vi "ActionVIOnRecompile.vi"(8 "error in":errorcluster, 9 "Timeout (ms)":u32, 10 "Runtime Configurable Section Path":string, 11 "Device Item Ref in":T1 format="%.0x") -> (0 "error out":errorcluster)   [LabVIEW 2026, in "Runtime Configuration Support Example System Explorer.lvlib"]
uses:
  Runtime Configuration Support Example System Explorer.lvlib
  <vilib>/NI VeriStand/Custom Device API/Custom Device Item Ref.ctl
  Shared/Compiled.Settings.ctl
  <vilib>/NI VeriStand/Custom Device API/Custom Device Channel Type.ctl
  <vilib>/NI VeriStand/Custom Device API/Data Access Type.ctl
  Error Constants.vi
  <vilib>/NI VeriStand/Execution/CustomDevice/NI VeriStand - Send Custom Device Message (Byte Array).vi
  <vilib>/NI VeriStand/Custom Device API/Custom Device API.lvlib
  <vilib>/NI VeriStand/Execution/CustomDevice/NI_VS Custom Device ExecutionAPI.lvlib
  Shared/Runtime Configuration Support Example Shared.lvlib
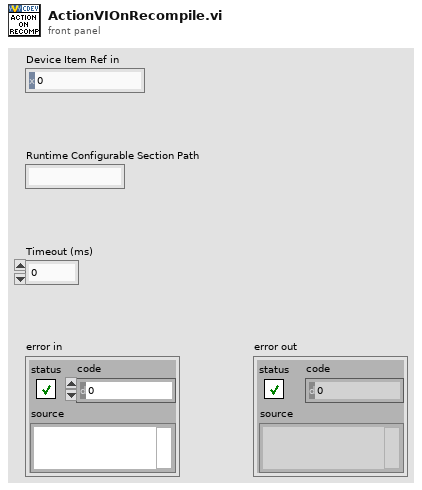
[diagram p1: front panel]
types:
  T1 = typedef "Custom Device API.lvlib/Custom Device Item Ref.ctl" = u64
  T2 = cluster{"Dynamic Config Status":bool, "Inports":i32[], "Outports":i32[], "Error":errorcluster}
  T3 = typedef "Custom Device API.lvlib/Custom Device Channel Type.ctl" = enum16{"Input", "Output"}
  T4 = typedef "Custom Device API.lvlib/Data Access Type.ctl" = enum16{"Read", "Write"}
  T5 = typedef "Runtime Configuration Support Example Shared.lvlib/Compiled.Settings.ctl" = cluster{"Name":string, "Inport SignalIDs":i32[], "Outport SignalIDs":i32[], "Inport Channel refs":T1[], "Outport Channel refs":T1[], "Inport Values":dbl[], "Outport Values":dbl[], "Device Error":errorcluster, "Dynamic Config Status":bool, "Response Ref":refnum<queue>}
  T6 = typedef "Custom Device API.lvlib/Custom Device Item Info.ctl" = cluster{"Name":string, "Is Channel":bool, "GUID":string, "Is Waveform":bool}
  T7 = typedef "Custom Device API.lvlib/Data Reference.ctl" = i32
  T8 = typedef "NI_VS Custom Device ExecutionAPI.lvlib/Custom Device Ref.ctl" = refnum<k24>
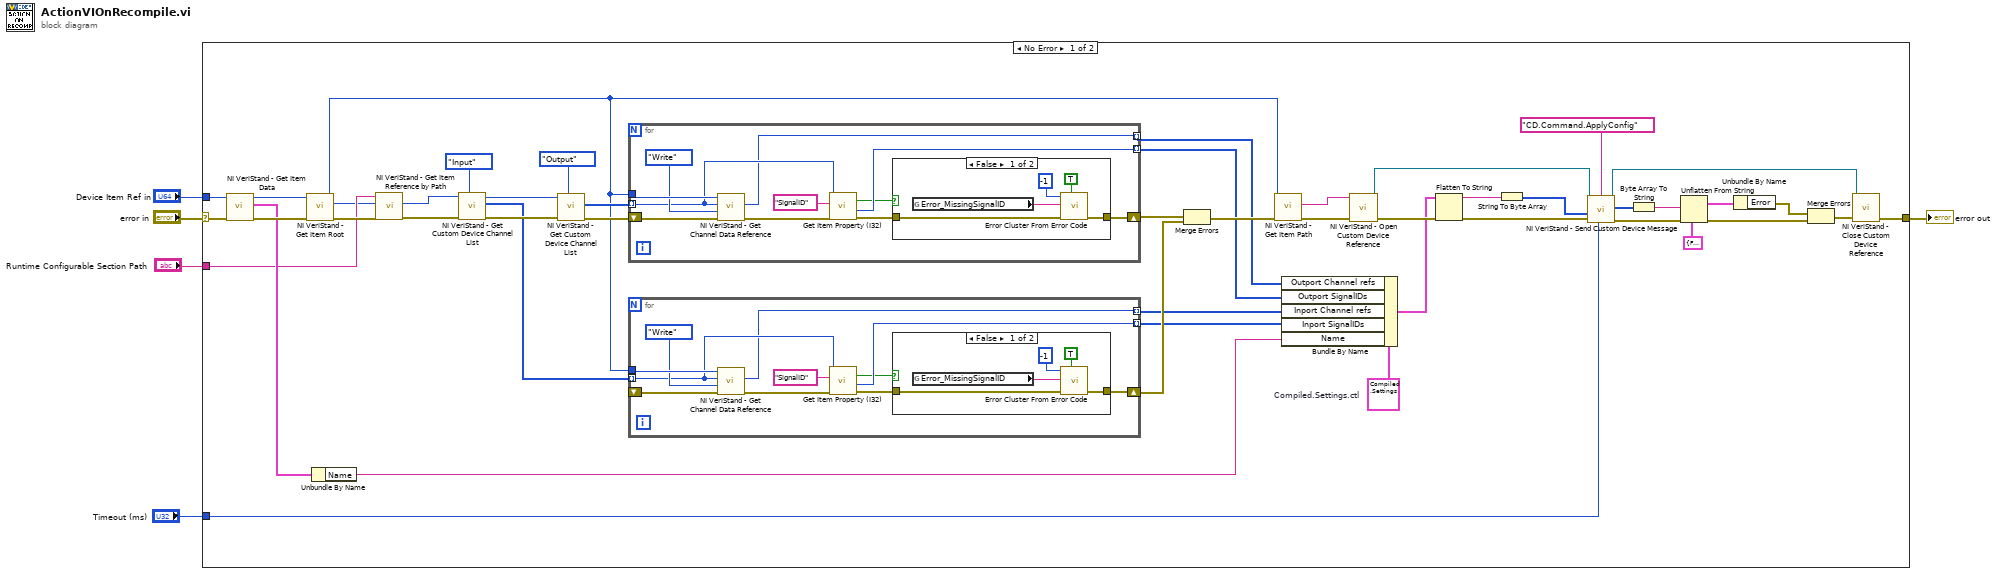
[diagram p0: block diagram]
diagram:
  n1 = case shown="No Error" "error in" {
    selector: "error in" -> [w52 w87]
    tunnel: [w43 w87] -> w4
    tunnel: "Device Item Ref in" -> [w35 _]
    tunnel: "Runtime Configurable Section Path" -> [w31 _]
    tunnel: "Timeout (ms)" -> [w20 _]
    frame No Error {
      w6 = T5 {"Name"="", "Inport SignalIDs"=[], "Outport SignalIDs"=[], "Inport Channel refs"=[], "Outport Channel refs"=[], "Inport Values"=[], "Outport Values"=[], "Device Error"={"status"=FALSE, "code"=0, "source"=""}, "Dynamic Config Status"=FALSE, "Response Ref"=refnum}  # Compiled.Settings.ctl
      n2 = call <vilib>:"NI VeriStand - Get Item Data.vi"("error in (no error)"=w52, "Item Ref in"=w35) -> ("error out"=w51:errorcluster, "Item Info"=w34:T6, "Item Ref out"=w32:T1)  [unwired: 6 in, 1 out]
      n3 = call <vilib>:"NI VeriStand - Get Item Root.vi"("error in (no error)"=w51, "Item Ref in"=w32) -> ("error out"=w50:errorcluster, "Root Ref out"=w30:T1, "Item Ref out"=w10:T1)  [unwired: 6 in, 1 out]
      n4 = Unbundle By Name(w34) -> ("Name"=w33:string)
      n5 = call <vilib>:"NI VeriStand - Get Item Reference by Path.vi"("error in (no error)"=w50, "Root Ref"=w30, "Item Path in"=w31) -> ("error out"=w49:errorcluster, "Item Ref"=w26:T1)  [unwired: 5 in, 2 out]
      n6 = call <vilib>:"NI VeriStand - Get Custom Device Channel List.vi"("Channel Type"=Custom_Device_Channel_Type."Input", "error in (no error)"=w49, "Device Ref in"=w26) -> ("error out"=w48:errorcluster, "Specified Channel Ref List"=w9:T1[], "Device Ref out"=w18:T1)  [unwired: 6 in]
      n7 = call <vilib>:"NI VeriStand - Get Custom Device Channel List.vi"("Channel Type"=Custom_Device_Channel_Type."Output", "error in (no error)"=w48, "Device Ref in"=w18) -> ("error out"=w47:errorcluster, "Specified Channel Ref List"=w28:T1[])  [unwired: 6 in, 1 out]
      n8 = for {
        tunnel: w28 -> [w74] mode=indexing
        shift-right: [w77] -> w37
        shift-left: w47 -> [w80]
        tunnel: w10 -> [w76]
        tunnel: [w72] -> w12 mode=indexing
        tunnel: [w71] -> w11 mode=indexing
        n9 = call <vilib>:"NI VeriStand - Get Channel Data Reference.vi"("error in (no error)"=w80, "Access"=Data_Access_Type."Write", "Channel Ref in"=w74, "Device Ref in"=w76) -> ("error out"=w79:errorcluster, "Channel Data Reference"=w72:T7)  [unwired: 5 in, 1 out]
        n10 = call <vilib>:"Get Item Property (I32).vi"("error in (no error)"=w79, "Property Name"="SignalID", "Item Ref in"=w74) -> ("error out"=w78:errorcluster, "Value"=w71:i32, "Found?"=w70:bool)  [unwired: 5 in, 1 out]
        n11 = case shown="False" w70 {
          tunnel: w78 -> [w85 w86]
          tunnel: [w84 w86] -> w77
          frame False {
            n12 = global read "Error Constants.vi" "Error_MissingSignalID"() -> (w82:string)
            n13 = call <vilib>:"Error Cluster From Error Code.vi"("show call chain? (False)"=TRUE, "error in (no error)"=w85, "error message (\"\")"=w82, "error code (0)"=-1) -> ("error out"=w84:errorcluster)  [unwired: 5 in]
          }
          frame True {
          }
        }
      }
      n14 = for {
        tunnel: w9 -> [w57] mode=indexing
        shift-right: [w60] -> w38
        shift-left: _ -> [w63]
        tunnel: w10 -> [w59]
        tunnel: [w55] -> w8 mode=indexing
        tunnel: [w54] -> w7 mode=indexing
        n15 = call <vilib>:"NI VeriStand - Get Channel Data Reference.vi"("error in (no error)"=w63, "Access"=Data_Access_Type."Write", "Channel Ref in"=w57, "Device Ref in"=w59) -> ("error out"=w62:errorcluster, "Channel Data Reference"=w55:T7)  [unwired: 5 in, 1 out]
        n16 = call <vilib>:"Get Item Property (I32).vi"("error in (no error)"=w62, "Property Name"="SignalID", "Item Ref in"=w57) -> ("error out"=w61:errorcluster, "Value"=w54:i32, "Found?"=w53:bool)  [unwired: 5 in, 1 out]
        n17 = case shown="False" w53 {
          tunnel: w61 -> [w68 w69]
          tunnel: [w67 w69] -> w60
          frame False {
            n18 = global read "Error Constants.vi" "Error_MissingSignalID"() -> (w65:string)
            n19 = call <vilib>:"Error Cluster From Error Code.vi"("show call chain? (False)"=TRUE, "error in (no error)"=w68, "error message (\"\")"=w65, "error code (0)"=-1) -> ("error out"=w67:errorcluster)  [unwired: 5 in]
          }
          frame True {
          }
        }
      }
      n20 = Merge Errors(w37, w38) -> (w36:errorcluster)
      n21 = call <vilib>:"NI VeriStand - Get Item Path.vi"("error in (no error)"=w36, "Item Ref in"=w10) -> ("error out"=w46:errorcluster, "Path"=w25:string)  [unwired: 6 in, 2 out]
      n22 = Bundle By Name(cluster=w6, "Outport Channel refs"=w12, "Outport SignalIDs"=w11, "Inport Channel refs"=w8, "Inport SignalIDs"=w7, "Name"=w33) -> (w24:T5)
      n23 = call <vilib>:"NI VeriStand - Open Custom Device Reference.vi"("error in (no error)"=w46, "Custom Device Path"=w25) -> ("error out"=w45:errorcluster, "Custom Device"=w19:T8)  [unwired: 8 in]
      n24 = Flatten To String(anything=w24, error in (no error)=w45) -> (data string=w23:string, error out=w44:errorcluster)  [unwired: 2 in, 1 out]
      n25 = String To Byte Array(string=w23) -> (unsigned byte array=w22:u8[])
      n26 = call-poly <vilib>:"NI VeriStand - Send Custom Device Message.vi"("Timeout ms (5000)"=w20, "error in (no error)"=w44, "Data"=w22, "Command"="CD.Command.ApplyConfig", "Custom Device in"=w19) -> ("error out"=w40:errorcluster, "Response"=w16:u8[], "Custom Device out"=w17:T8)  [unwired: 4 in]
      n27 = Byte Array To String(unsigned byte array=w16) -> (string=w15:string)
      n28 = Unflatten From String(type=T2 {"Dynamic Config Status"=FALSE, "Inports"=[], "Outports"=[], "Error"={"status"=FALSE, "code"=0, "source"=""}}, binary string=w15, error in (no error)=w40) -> (value=w14:T2, error out=w39:errorcluster)  [unwired: 2 in, 1 out]
      n29 = Unbundle By Name(w14) -> ("Error"=w41:errorcluster)
      n30 = Merge Errors(w41, w39) -> (w42:errorcluster)
      n31 = call <vilib>:"NI VeriStand - Close Custom Device Reference.vi"("error in (no error)"=w42, "Custom Device"=w17) -> ("error out"=w43:errorcluster)  [unwired: 9 in]
    }
    frame Error {
    }
  }
  "error out" <- w4
